vi "RX-SIS-SIM-UDP.vi"() -> ()   [LabVIEW 2017]
uses:
  <vilib>/Platform/TimedLoop/XDataNode/timing_clust.ctl
  <vilib>/Platform/TimedLoop/XDataNode/nitl_modes.ctl
  <vilib>/Platform/TimedLoop/XDataNode/wakeup.ctl
  <vilib>/Platform/TimedLoop/XDataNode/XDataNode.xnode
  <vilib>/Platform/TimedLoop/XDataNode/XDNodeRunTimeDep.lvlib
panel:
  in  "Stop":bool
  out "SIS-SIM-RX-ARRAY":dbl[](array[numeric])
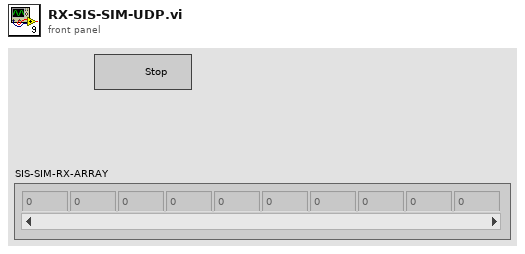
[diagram p1: front panel]
types:
  T1 = typedef "XDNodeRunTimeDep.lvlib/timing_clust.ctl" = cluster{"Expected End [f-1]":u64, "Actual End [f-1]":u64, "Finished Late? [f-1]":bool, "Expected End [i-1]":u64, "Actual End [i-1]":u64, "Finished Late? [i-1]":bool, "Expected Start [i]":u64, "Actual Start [i]":u64, "Expected Start [f]":u64, "Actual Start [f]":u64, "Source Name":string, "Structure Name":string, "Period":i64, "Deadline":i64, "Offset":i64, "Start":i64, "Priority":i32, "Timeout":i32, "Mode":T2, "Wakeup Reason":T3, "Error":errorcluster, "Source Type":string, "Secondary Source Type":string, "Global End Time":u64, "Global Start Time":u64, "Frame Duration":u64, "Iteration Duration":u64, "Assigned CPU":i32, "I/O Scan Engine Mode":u32}
  T2 = typedef "XDNodeRunTimeDep.lvlib/nitl_modes.ctl" = enum32{"No Change", "Process missed periods, maintain original phase", "Discard missed periods, maintain original phase", "Process missed periods, ignore original phase", "Discard missed periods, ignore original phase"}
  T3 = typedef "XDNodeRunTimeDep.lvlib/wakeup.ctl" = enum32{"Normal", "Aborted", "Asynchronous wakeup", "Timing source error", "Timed loop error", "Timeout"}
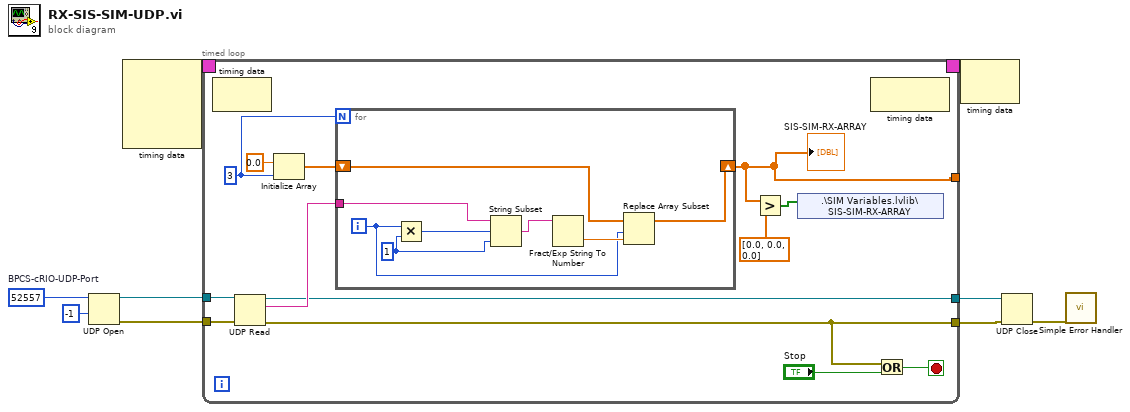
[diagram p0: block diagram]
diagram:
  w7 = u16 52557  # BPCS-cRIO-UDP-Port
  n1 = UDP Open(9:-1 ("timeout ms (25000)"), 11:w7) -> (port=w6:refnum<k16>, 0:w5:errorcluster)  [unwired: 3 in, 1 out]
  n2 = node-c288() -> (w9:T1)  [unwired: 4 in]
  n3 = timed-loop {
    timing: w9 -> [_]
    timing-out: [_] -> w8
    tunnel: w6 -> [w20]
    tunnel: w5 -> [w19]
    tunnel: [w17] -> w3
    tunnel: [w16] -> w2
    tunnel: [w12] -> _
    stop <- w21 stop-if-true
    w13 = 3 ("dimension size")
    n4 = node-c288() -> ()  [unwired: 1 in, 1 out]
    n5 = UDP Read(connection ID=w20, 8:w19) -> (data out=w18:string, error out=w16:errorcluster, 3:w17:refnum<k16>)  [unwired: 1 in, 3 out]
    n6 = Initialize Array(0.0 ("element"), w13) -> (w14:dbl[])
    n7 = for {
      N: w13 -> [_]
      tunnel: w18 -> [w29]
      shift-right: [w25] -> w12
      shift-left: w14 -> [w24]
      i -> [w26]
      w23 = 1 ("y")
      n8 = Multiply(x=w26, y=w23) -> (x*y=w28:i32)
      n9 = String Subset(string=w29, offset (0)=w28, length (rest)=w23) -> (substring=w30:string)
      n10 = Fract/Exp String To Number(string=w30) -> (number=w27:dbl)  [unwired: 3 in, 1 out]
      n11 = Replace Array Subset(array=w24, new element=w27, index=w26) -> (w25:dbl[])
    }
    "SIS-SIM-RX-ARRAY" <- w12
    n12 = Greater?(x=w12, y=dbl[] [0.0, 0.0, 0.0]) -> (0:w10:bool[])
    n13 = shared-variable ".\\SIM Variables.lvlib\\SIS-SIM-RX-ARRAY"(w10) -> ()  [unwired: 1 in, 1 out]
    n14 = node-c288() -> ()  [unwired: 1 in, 1 out]
    n15 = Or(x=w16, y="Stop") -> (x .or. y?=w21:bool)
  }
  n16 = node-c288(w8) -> ()  [unwired: 1 out]
  n17 = UDP Close(connection ID=w3, 8:w2) -> (error out=w4:errorcluster)  [unwired: 1 out]
  n18 = call <vilib>:"Simple Error Handler.vi"("error in (no error)"=w4) -> ()  [unwired: 4 in, 5 out]
